vi "GE5565 DMA Write Interrupt (U8).vi"(6 "timeout (1000 ms)":u32=1000, 8 "error in (no error)":errorcluster, 9 "buffer":u8[](array[numeric]), 10 "offset (0)":u32, 11 "VMIC reference in":T1) -> (0 "error out":errorcluster, 3 "VMIC reference out":T1, 5 "Times":cluster{u32, u32})   [LabVIEW 2016]
uses:
  <vilib>/Instr/_visa.llb/Select Event Type.ctl
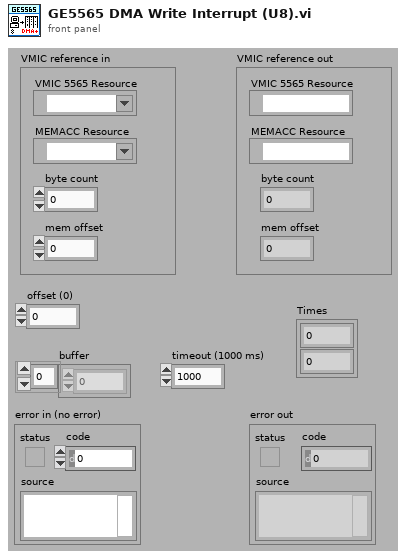
[diagram p1: front panel]
types:
  T1 = cluster{"VMIC 5565 Resource":refnum<visa-resource-name>, "MEMACC Resource":refnum<visa-resource-name>, "byte count":u32, "mem offset":u32}
  T2 = typedef "Select Event Type.ctl" = u32
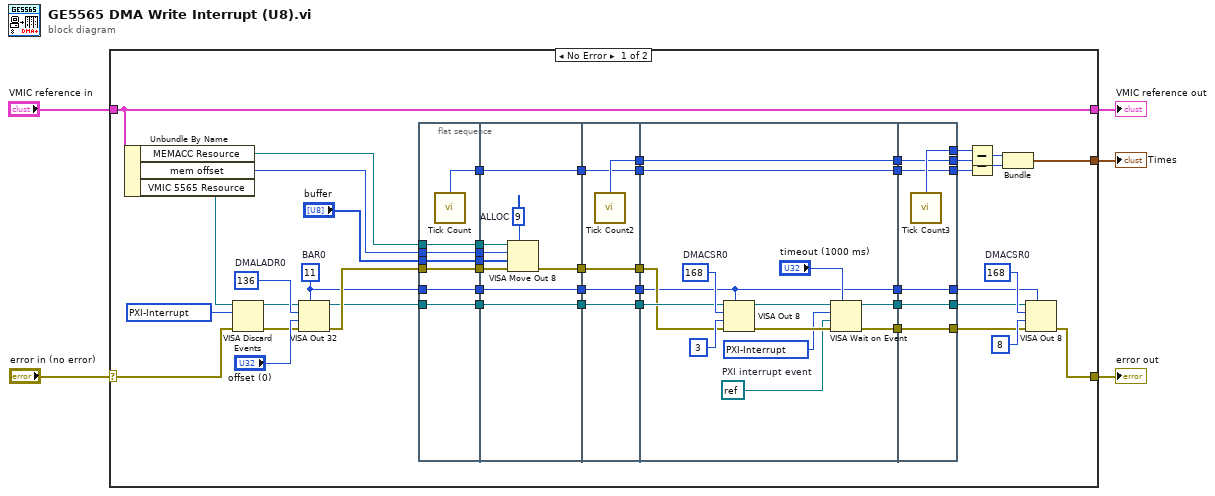
[diagram p0: block diagram]
diagram:
  n1 = case shown="No Error" "error in (no error)" {
    selector: "error in (no error)" -> [w50 w94]
    tunnel: "VMIC reference in" -> [w41 w95]
    tunnel: [w41 w95] -> w2
    tunnel: [w38 w94] -> w4
    tunnel: [w6 _] -> w1
    frame No Error {
      w36 = u16 11  # BAR0
      w40 = u32 168  # DMACSR0
      w47 = T2 1073684514 items=["ServiceRequest"=1073684491, "Trigger"=3221168138, "Clear"=1073684493, "VXI-Signal"=1073684512, "VXI/VME-Interrupt"=3221168161, "VXI/VME-Sysfail"=1073684509, "VXI/VME-Sysreset"=1073684510, "GPIB-CIC"=1073684498, "GPIB-Talk"=1073684499, "GPIB-Listen"=1073684500, "PXI-Interrupt"=1073684514, "AllEnabled"=1073709055] ("Event Type")
      w52 = u32 136  # DMALADR0
      n2 = Unbundle By Name(w41) -> ("MEMACC Resource"=w42:refnum<visa-resource-name>, "mem offset"=w43:u32, "VMIC 5565 Resource"=w45:refnum<visa-resource-name>)
      n3 = VISA Discard Events(8:w50, 10:w47, 11:w45) -> (0:w48:errorcluster, 3:w49:refnum<visa-resource-name>)  [unwired: 1 in]
      n4 = VISA Out 32(7:w36, 8:w48, 9:"offset (0)", 10:w52, 11:w49) -> (0:w44:errorcluster, 3:w37:refnum<visa-resource-name>)
      n5 = flat-sequence {
        tunnel: w36 -> [w54]
        tunnel: w37 -> [w55]
        tunnel: w42 -> [w56]
        tunnel: w43 -> [w57]
        tunnel: w44 -> [w58]
        tunnel: "buffer" -> [w59]
        tunnel: [w59] -> w32
        tunnel: [w58] -> w31
        tunnel: [w57] -> w30
        tunnel: [w56] -> w29
        tunnel: [w55] -> w28
        tunnel: [w54] -> w27
        tunnel: [w53] -> w12
        tunnel: [w66] -> w35
        tunnel: [w62] -> w34
        tunnel: [w61] -> w33
        tunnel: w32 -> [w67]
        tunnel: w31 -> [w65]
        tunnel: w30 -> [w64]
        tunnel: w29 -> [w63]
        tunnel: w28 -> [w62]
        tunnel: w27 -> [w61]
        tunnel: [w60] -> w13
        tunnel: w12 -> [w60]
        tunnel: w35 -> [w73]
        tunnel: w34 -> [w72]
        tunnel: w33 -> [w71]
        tunnel: [w73] -> w26
        tunnel: [w72] -> w25
        tunnel: [w71] -> w24
        tunnel: [w70] -> w16
        tunnel: [w69] -> w14
        tunnel: w13 -> [w69]
        tunnel: w26 -> [w78]
        tunnel: w25 -> [w80]
        tunnel: w24 -> [w76]
        tunnel: [w79] -> w20
        tunnel: [w76] -> w19
        tunnel: [w77] -> w18
        tunnel: [w75] -> w17
        tunnel: w16 -> [w75]
        tunnel: [w74] -> w15
        tunnel: w14 -> [w74]
        tunnel: [w91] -> w21
        tunnel: [w92] -> w23
        tunnel: [w93] -> w22
        tunnel: w20 -> [w93]
        tunnel: w19 -> [w92]
        tunnel: w18 -> [w91]
        tunnel: [w90] -> w11
        tunnel: [w89] -> w10
        tunnel: w17 -> [w89]
        tunnel: w15 -> [w88]
        tunnel: [w88] -> w9
        frame #0 {
          n6 = call "Tick Count"() -> ("Tick Count(uSec)"=w53:u32)
        }
        frame #1 {
          w68 = u16 9  # ALLOC
          n7 = VISA Move Out 8(7:w68, 8:w65, 9:w67, 10:w64, 11:w63) -> (0:w66:errorcluster)  [unwired: 1 out]
        }
        frame #2 {
          n8 = call "Tick Count2"() -> ("Tick Count(uSec)"=w70:u32)
        }
        frame #3 {
          w85 = refnum<visa-resource-name> refnum  # PXI interrupt event
          w84 = T2 1073684514 items=["ServiceRequest"=1073684491, "Trigger"=3221168138, "Clear"=1073684493, "VXI-Signal"=1073684512, "VXI/VME-Interrupt"=3221168161, "VXI/VME-Sysfail"=1073684509, "VXI/VME-Sysreset"=1073684510, "GPIB-CIC"=1073684498, "GPIB-Talk"=1073684499, "GPIB-Listen"=1073684500, "PXI-Interrupt"=1073684514, "AllEnabled"=1073709055] ("Event Type")
          w81 = u32 168  # DMACSR0
          n9 = VISA Out 8(7:w76, 8:w78, 9:u8 3 ("value (0)"), 10:w81, 11:w80) -> (0:w87:errorcluster, 3:w86:refnum<visa-resource-name>)
          n10 = VISA Wait on Event(7:"timeout (1000 ms)", 8:w87, 9:w85, 10:w84, 11:w86) -> (0:w77:errorcluster, 3:w79:refnum<visa-resource-name>)  [unwired: 2 out]
        }
        frame #4 {
          n11 = call "Tick Count3"() -> ("Tick Count(uSec)"=w90:u32)
        }
      }
      n12 = Subtract(x=w11, y=w10) -> (x-y=w8:u32)
      n13 = Subtract(x=w10, y=w9) -> (x-y=w7:u32)
      n14 = Bundle(w8, w7) -> (w6:cluster{u32, u32})  [unwired: 1 in]
      n15 = VISA Out 8(7:w23, 8:w21, 9:u8 8 ("value (0)"), 10:w40, 11:w22) -> (0:w38:errorcluster)  [unwired: 1 out]
    }
    frame Error {
    }
  }
  "error out" <- w4
  "VMIC reference out" <- w2
  "Times" <- w1
